vi "Read Positions.vi"(8 "error in (no error)":errorcluster, 11 "Port In":T3={"P type"=0, "reference"="", " Terminator "="\r\n", "Timeout"=300} {"Timeout" step=10; "P type" items=["none", "RS-232C"]}) -> (0 "error out":errorcluster, 1 "Calculated Position":T2, 2 "Encoder Position":T1, 3 "Port Out":T3={"P type"=0, "reference"="", " Terminator "="\r\n", "Timeout"=300} {"Timeout" step=10; "P type" items=["none", "RS-232C"]})   [LabVIEW 2021]
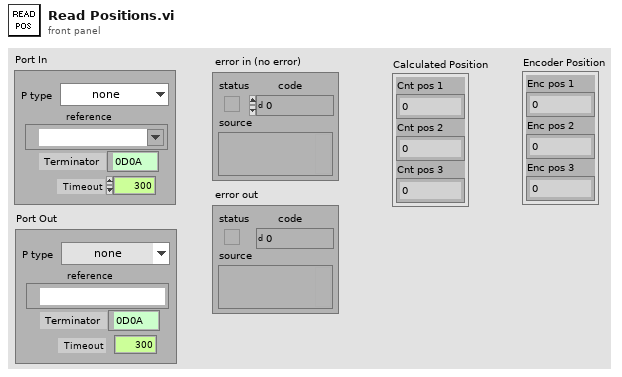
[diagram p1: front panel]
types:
  T1 = cluster{"Enc pos 1":dbl, "Enc pos 2":dbl, "Enc pos 3":dbl}
  T2 = cluster{"Cnt pos 1":dbl, "Cnt pos 2":dbl, "Cnt pos 3":dbl}
  T3 = cluster{"P type":u16, "reference":refnum<visa-resource-name>, " Terminator ":string, "Timeout":i32}
  T4 = cluster{"Enc pos":dbl, "Enc pos":dbl, "Enc pos":dbl}
  T5 = cluster{"Cnt pos":dbl, "Cnt pos":dbl, "Cnt pos":dbl}
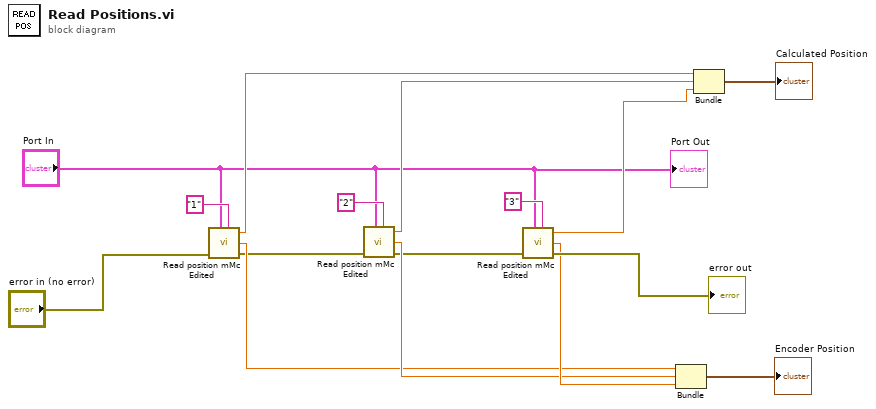
[diagram p0: block diagram]
diagram:
  n1 = call "Read position mMc Edited.vi"("Port"="Port In", "error in (no error)"="error in (no error)", "Controller #"="1") -> ("Cnt pos"=w10:dbl, "Enc pos"=w6:dbl, "error out"=w2:errorcluster)  [unwired: 4 in]
  n2 = call "Read position mMc Edited.vi"("Port"="Port In", "error in (no error)"=w2, "Controller #"="2") -> ("Cnt pos"=w11:dbl, "Enc pos"=w7:dbl, "error out"=w3:errorcluster)  [unwired: 4 in]
  n3 = call "Read position mMc Edited.vi"("Port"="Port In", "error in (no error)"=w3, "Controller #"="3") -> ("Cnt pos"=w12:dbl, "Enc pos"=w8:dbl, "error out"=→"error out":errorcluster)  [unwired: 4 in]
  n4 = Bundle("Enc pos"=w6, "Enc pos"=w7, "Enc pos"=w8) -> (→"Encoder Position":T4)  [unwired: 1 in]
  n5 = Bundle("Cnt pos"=w10, "Cnt pos"=w11, "Cnt pos"=w12) -> (→"Calculated Position":T5)  [unwired: 1 in]
  "Port Out" <- "Port In"
